vi "UpdateList.vi"(4 "Fitted Circle (Find Circular Edge 1)":T1 {"Average SNR (dB)" format="%.2f"; "Average Strength" format="%.2f"; "Roundness (Real-World)" format="%.2f"; "Radius (Real-World)" format="%.2f"; "Center (Real-World)"."Y" format="%.2f"; "Center (Real-World)"."X" format="%.2f"; "Radius (Pixels)" format="%.2f"; "Center (Pixels)"."Y" format="%.2f"; "Center (Pixels)"."X" format="%.2f"}, 6 "Matches":T3(array[cluster]) {"Bounding Box"."y" format="%.2f"; "Bounding Box"."x" format="%.2f"; "Position"."y" format="%.2f"; "Position"."x" format="%.2f"; "Score" format="%.2f"; "Scale" format="%.2f"; "Angle" format="%.2f"}, 8 "错误输入":errorcluster, 10 "MCListbox引用句柄":refnum<vi>, 11 "Image in":T2(plugin-control)) -> (0 "错误输出":errorcluster, 3 "Image out":T2(plugin-control))   [LabVIEW 2016]
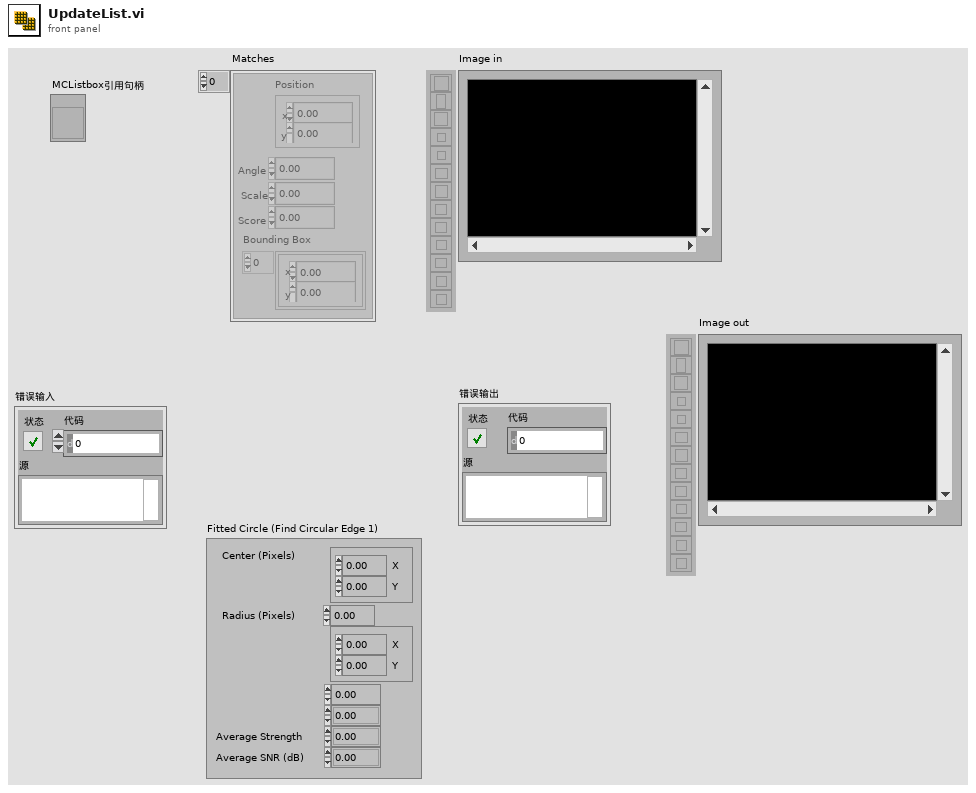
[diagram p1: front panel]
types:
  T1 = cluster{"Center (Pixels)":cluster{"X":sgl, "Y":sgl}, "Radius (Pixels)":dbl, "Center (Real-World)":cluster{"X":sgl, "Y":sgl}, "Radius (Real-World)":dbl, "Roundness (Real-World)":dbl, "Average Strength":dbl, "Average SNR (dB)":dbl}
  T2 = typedef "IMAQ Image.ctl" = refnum<image>
  T3 = cluster{"Position":cluster{"x":sgl, "y":sgl}, "Angle":sgl, "Scale":sgl, "Score":sgl, "Bounding Box":cluster{"x":sgl, "y":sgl}[]}[]
  T4 = typedef "IMAQ Circle" = cluster{"Center X":i32, "Center Y":i32, "Inner Radius":i32, "Outer Radius":i32, "Start Angle":dbl, "End Angle":dbl}
  T5 = cluster{"Position":cluster{"x":sgl, "y":sgl}, "Angle":sgl, "Scale":sgl, "Score":sgl, "Bounding Box":cluster{"x":sgl, "y":sgl}[]}
  T6 = typedef "ROI Descriptor" = cluster{"Global Rectangle":i32[], "Contours":cluster{"ID":enum32{"External", "Internal"}, "Type":u32, "Coordinates":i32[]}[]}
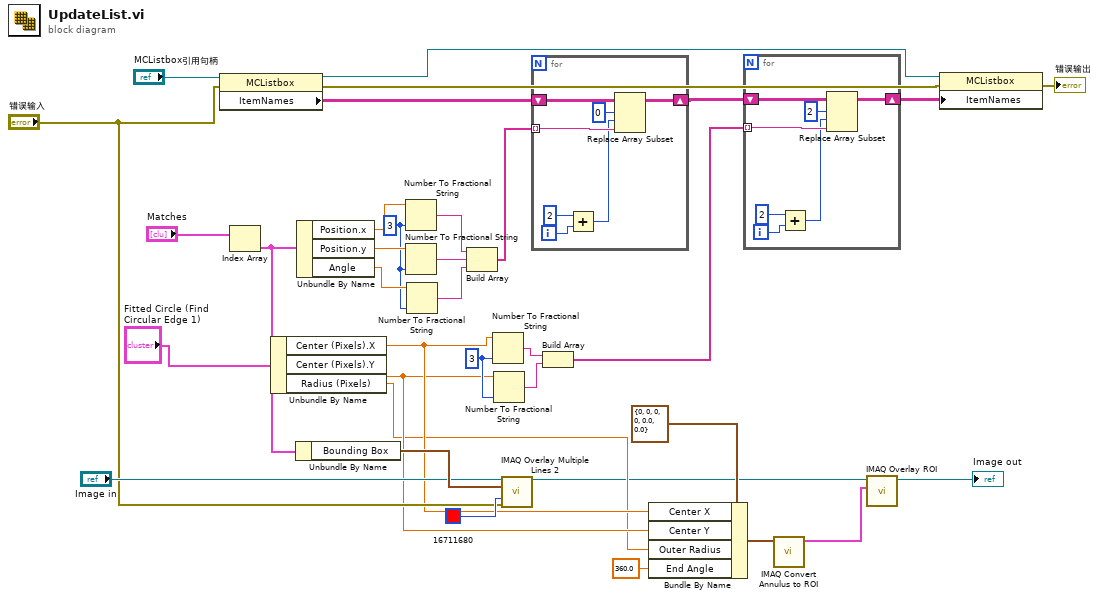
[diagram p0: block diagram]
diagram:
  w16 = i16 3 ("精度(6)")
  w17 = i16 3 ("精度(6)")
  n1 = property class="MCListbox"(reference="MCListbox引用句柄", error in="错误输入") -> (reference out=w20:refnum<vi>, error out=w19:errorcluster, "ItemNames"=w34:string[][])
  n2 = Index Array(array="Matches") -> (element=w15:T5)  [unwired: 1 in]
  n3 = Unbundle By Name("Fitted Circle (Find Circular Edge 1)") -> ("Center (Pixels).X"=w9:sgl, "Center (Pixels).Y"=w8:sgl, "Radius (Pixels)"=w7:dbl)
  n4 = Unbundle By Name(w15) -> ("Bounding Box"=w14:cluster{"x":sgl, "y":sgl}[])
  n5 = Unbundle By Name(w15) -> ("Position.x"=w32:sgl, "Position.y"=w31:sgl, "Angle"=w30:sgl)
  n6 = Number To Fractional String(number=w32, precision (6)=w17) -> (F-format string=w29:string)  [unwired: 2 in]
  n7 = Number To Fractional String(number=w31, precision (6)=w17) -> (F-format string=w28:string)  [unwired: 2 in]
  n8 = Number To Fractional String(number=w30, precision (6)=w17) -> (F-format string=w27:string)  [unwired: 2 in]
  n9 = Build Array(w29, w28, w27) -> (w26:string[])
  n10 = Number To Fractional String(number=w9, precision (6)=w16) -> (F-format string=w25:string)  [unwired: 2 in]
  n11 = Number To Fractional String(number=w8, precision (6)=w16) -> (F-format string=w24:string)  [unwired: 2 in]
  n12 = call "IMAQ Overlay Multiple Lines 2"("Image"="Image in", "Line End Points"=w14, "Color"=u32 16711680, "error in (no error)"="错误输入") -> ("Image Out"=w3:T2)  [unwired: 10 in, 1 out]
  n13 = for {
    shift-right: [w40] -> w22
    shift-left: w34 -> [w42]
    tunnel: w26 -> [w39] mode=indexing
    i -> [w38]
    n14 = Add(x=2, y=w38) -> (x+y=w36:i32)
    n15 = Replace Array Subset(array=w42, new element=w39, index (row)=0 ("索引 (行)"), index (col)=w36) -> (w40:string[][])
  }
  n16 = Build Array(w25, w24) -> (w23:string[])
  n17 = Bundle By Name(cluster=T4 {"Center X"=0, "Center Y"=0, "Inner Radius"=0, "Outer Radius"=0, "Start Angle"=0.0, "End Angle"=0.0} ("Annulus"), "Center X"=w9, "Center Y"=w8, "Outer Radius"=w7, "End Angle"=360.0) -> (w5:T4)
  n18 = for {
    shift-right: [w47] -> w21
    shift-left: w22 -> [w49]
    tunnel: w23 -> [w46] mode=indexing
    i -> [w45]
    n19 = Add(x=2, y=w45) -> (x+y=w43:i32)
    n20 = Replace Array Subset(array=w49, new element=w46, index (row)=2 ("索引 (行)"), index (col)=w43) -> (w47:string[][])
  }
  n21 = call "IMAQ Convert Annulus to ROI"("Annulus"=w5) -> ("ROI Descriptor"=w4:T6)  [unwired: 8 in, 1 out]
  n22 = call "IMAQ Overlay ROI"("ROI Descriptor"=w4, "Image"=w3) -> ("Image Out"=→"Image out":T2)  [unwired: 8 in, 1 out]
  n23 = property class="MCListbox"(reference=w20, error in=w19, "ItemNames"=w21) -> (error out=→"错误输出":errorcluster)  [unwired: 1 out]
